vi "Main.vi"() -> ()   [LabVIEW 2020]
uses:
  894af00f-5b5e-4956-bdd0-dbfe7de3cfd1.vi
  2f02bd1a-2950-4099-aa5b-b00aa924ff99.vi
  6b85a64f-4064-4cca-92da-147d7fd17ded.vi
  3defe9b0-9a24-46bd-983e-5b9eb35e9ab3.vi
  b02ec4f8-b8d1-4e8f-904a-19f02c8769a2.vi
  fd6a9062-ef78-4eef-ac77-1a2b6e1554ba.vi
panel:
  in  "文字Y座標":dbl(slide)=0.08450704225352113
  in  "文字X座標":dbl(slide)=0.05384615384615385 scale=0.0..1.0
  in  "字體":string(combo)="微軟正黑體"
  in  "自動刷新桌布":bool
  in  "set wallpaper":bool
  in  "save png":bool
  in  "字體顏色":u32(colorbox)
  in  "背景顏色":u32(colorbox)=16777225
  in  "高":u16=1080
  in  "寬":u16=1920
  out "產生圖片":picture
  in  "文字設定":T1={"大小"=72, "刪除線"=FALSE, "斜體"=FALSE, "底線"=FALSE, "外線"=FALSE, "陰影"=FALSE, "粗體"=FALSE}
  in  "文字內容":string="學校簡稱:君毅中學\n科系名稱:資訊科\n崗位號碼:XX\n選手姓名:XXX"
  # "Poewered By CISH Networking Team"
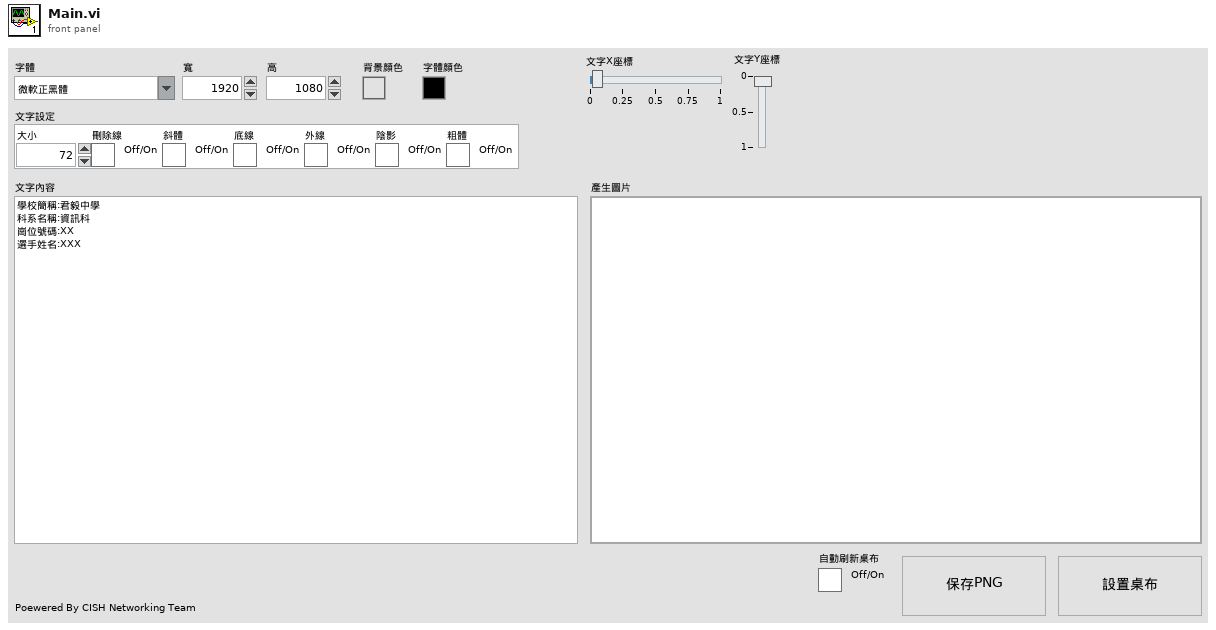
[diagram p1: front panel]
types:
  T1 = cluster{"大小":i16, "刪除線":bool, "斜體":bool, "底線":bool, "外線":bool, "陰影":bool, "粗體":bool}
  T2 = cluster{"left":i16, "top":i16, "right":i16, "bottom":i16}
  T3 = enum16{"User-specified Font", "Application Font", "System Font", "Dialog Font"}
  T4 = cluster{"Font Name:":string, "Size":i16, "Strikeout?":bool, "Italic?":bool, "Underline?":bool, "Outline?":bool, "Shadow?":bool, "Bold?":bool}
  T5 = typedef "imagedata.ctl" = cluster{"image type":i32, "image depth":i32, "image":u8[], "mask":u8[], "colors":u32[], "Rectangle":cluster{"left":i16, "top":i16, "right":i16, "bottom":i16}}
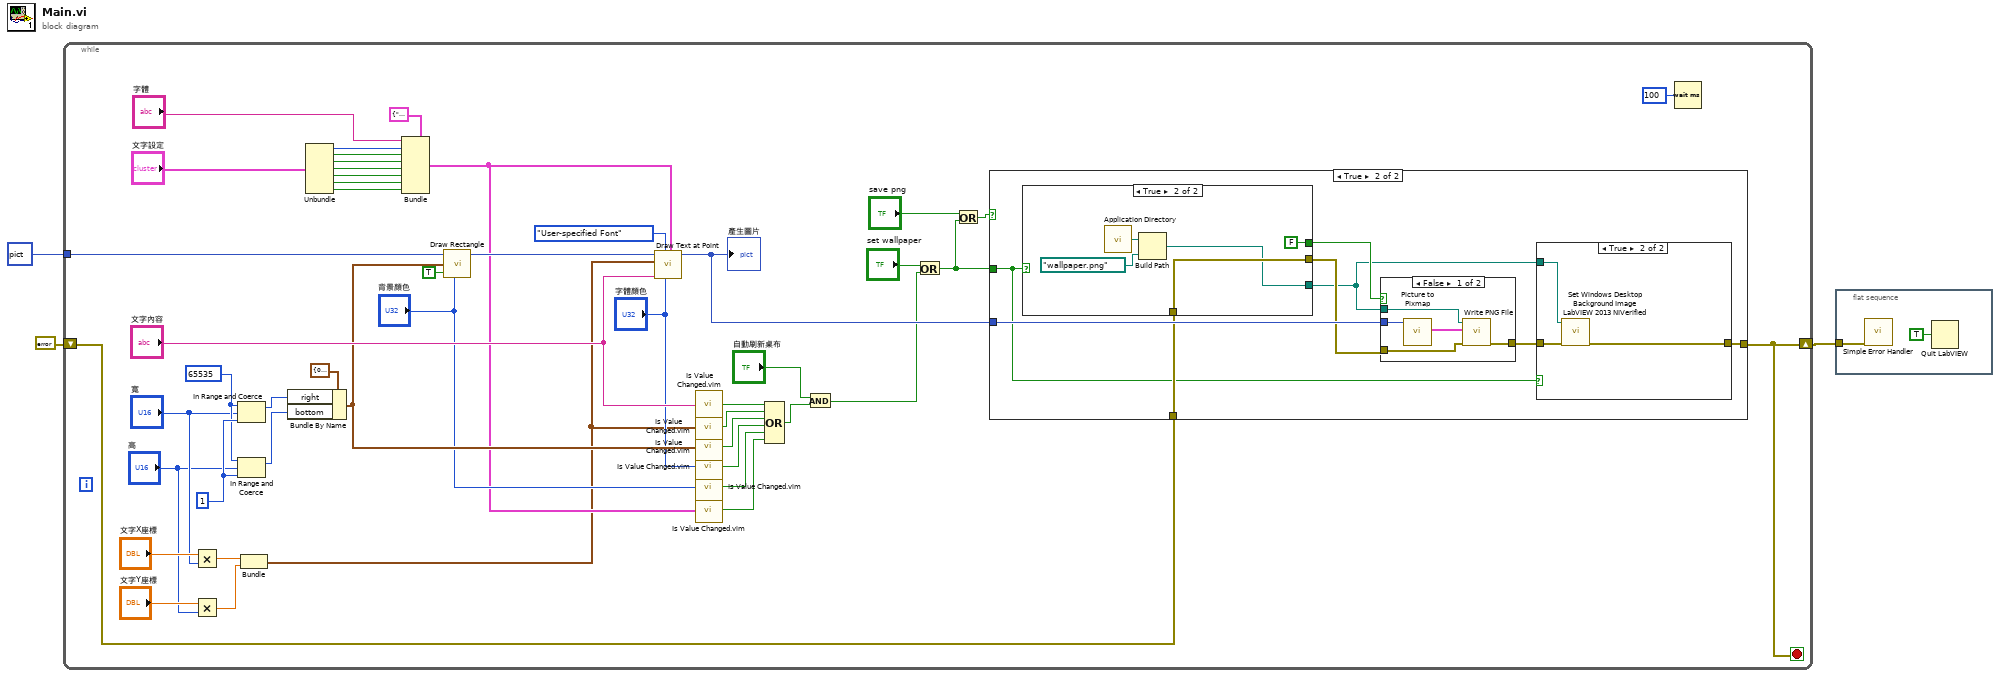
[diagram p0: block diagram]
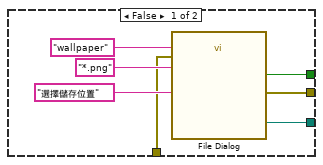
[diagram p4: hidden frame]
diagram:
  n1 = while {
    tunnel: picture data[5B] ("picture") -> [w42]
    shift-right: [w35] -> w1
    shift-left: errorcluster {"status"=FALSE, "code"=0, "source"=""} ("error out") -> [w36]
    stop <- w35 stop-if-true
    w24 = u16 65535 ("upper limit")
    w27 = u16 1 ("lower limit")
    n2 = Multiply(x="文字X座標", y="寬") -> (x*y=w6:dbl)
    n3 = Multiply(x="文字Y座標", y="高") -> (x*y=w5:dbl)
    n4 = In Range and Coerce(upper limit=w24, x="寬", lower limit=w27) -> (coerced(x)=w26:u16)  [unwired: 1 out]
    n5 = In Range and Coerce(upper limit=w24, x="高", lower limit=w27) -> (coerced(x)=w25:u16)  [unwired: 1 out]
    n6 = Bundle(w6, w5) -> (w4:cluster{dbl, dbl})  [unwired: 1 in]
    n7 = Bundle By Name(cluster=T2 {"left"=0, "top"=0, "right"=0, "bottom"=0} ("rect"), "right"=w26, "bottom"=w25) -> (w23:T2)
    n8 = Unbundle("文字設定") -> ("大小"=w49:i16, "刪除線"=w48:bool, "斜體"=w47:bool, "底線"=w46:bool, "外線"=w45:bool, "陰影"=w44:bool, "粗體"=w43:bool)
    n9 = Bundle(cluster=T4 {"Font Name:"="", "Size"=12, "Strikeout?"=FALSE, "Italic?"=FALSE, "Underline?"=FALSE, "Outline?"=FALSE, "Shadow?"=FALSE, "Bold?"=FALSE} ("[user-specified font]"), "Font Name:"="字體", "Size"=w49, "Strikeout?"=w48, "Italic?"=w47, "Underline?"=w46, "Outline?"=w45, "Shadow?"=w44, "Bold?"=w43) -> (w14:T4)
    n10 = call <vilib>:"Draw Rectangle.vi"("picture"=w42, "rect"=w23, "fill?(F)"=TRUE, "color(black)"="背景顏色") -> ("new picture"=w41:picture)  [unwired: 5 in]
    n11 = call <vilib>:"Draw Text at Point.vi"("[user-specified font]"=w14, "text color(black)"="字體顏色", "desired font(Application)"=T3."User-specified Font", "text"="文字內容", "origin"=w4, "picture"=w41) -> ("new picture"=w37:picture)  [unwired: 4 in, 1 out]
    "產生圖片" <- w37
    n12 = call "Is Value Changed.vim"("value"="文字內容") -> ("changed or first call?"=w20:bool)
    n13 = call "Is Value Changed.vim"("value"=w4) -> ("changed or first call?"=w19:bool)
    n14 = call "Is Value Changed.vim"("value"=w23) -> ("changed or first call?"=w18:bool)
    n15 = call "Is Value Changed.vim"("value"="字體顏色") -> ("changed or first call?"=w17:bool)
    n16 = call "Is Value Changed.vim"("value"="背景顏色") -> ("changed or first call?"=w16:bool)
    n17 = call "Is Value Changed.vim"("value"=w14) -> ("changed or first call?"=w13:bool)
    n18 = Compound Arithmetic op=OR(w20, w19, w18, w17, w16, w13) -> (w15:bool)
    n19 = And(x="自動刷新桌布", y=w15) -> (x .and. y?=w28:bool)
    n20 = Or(x="set wallpaper", y=w28) -> (x .or. y?=w11:bool)
    n21 = Or(x="save png", y=w11) -> (x .or. y?=w33:bool)
    n22 = case shown="True" w33 {
      tunnel: w37 -> [_ w60]
      tunnel: [w52 w53] -> w35
      tunnel: w36 -> [w52 w58]
      tunnel: w11 -> [_ w55]
      frame False {
      }
      frame True {
        n23 = case shown="True" w55 {
          tunnel: [w68 FALSE ("cancelled")] -> w59
          tunnel: [w67 w73] -> w54
          tunnel: w58 -> [w66 w76]
          tunnel: [w65 w76] -> w57
          frame False {
            n24 = call "File Dialog"("prompt"="選擇儲存位置", "default name"="wallpaper", "error in"=w66, "pattern (all files)"="*.png") -> ("selected path"=w67:path, "cancelled"=w68:bool, "error out"=w65:errorcluster)  [unwired: 8 in, 1 out]
          }
          frame True {
            n25 = call <vilib>:"Application Directory.vi"() -> ("Application Directory"=w72:path)
            n26 = Build Path(base path=w72, name or relative path=path "wallpaper.png") -> (appended path=w73:path)
          }
        }
        n27 = case shown="False" w59 {
          tunnel: w60 -> [w81 _]
          tunnel: w54 -> [w79 _]
          tunnel: [w78 _] -> w56
          tunnel: w57 -> [w77 _]
          frame False {
            n28 = call <vilib>:"Picture to Pixmap.vi"("picture"=w81) -> ("image data"=w80:T5)  [unwired: 9 in, 1 out]
            n29 = call <vilib>:"Write PNG File.vi"("error in (no error)"=w77, "image data"=w80, "path to PNG file"=w79) -> ("error out"=w78:errorcluster)  [unwired: 7 in, 1 out]
          }
          frame True {
          }
        }
        n30 = case shown="True" w55 {
          tunnel: w56 -> [w61 w64]
          tunnel: w54 -> [_ w63]
          tunnel: [w61 w62] -> w53
          frame False {
          }
          frame True {
            n31 = call "Set Windows Desktop Background Image LabVIEW 2013 NIVerified.vi"("error in (no error)"=w64, "Path"=w63) -> ("error out"=w62:errorcluster)  [unwired: 9 in]
          }
        }
      }
    }
    n32 = Wait (ms)(milliseconds to wait=u32 100) -> ()  [unwired: 1 out]
  }
  n33 = flat-sequence {
    tunnel: w1 -> [w83]
    frame #0 {
      n34 = call <vilib>:"Simple Error Handler.vi"("error in (no error)"=w83) -> ()  [unwired: 4 in, 5 out]
      n35 = Quit LabVIEW(quit? (T)=TRUE) -> ()
    }
  }
